vi "Remove Attribute - Many.vi"(8 "error in (no error)":errorcluster, 10 "Attributes":string[](array[string]), 11 "YAML Parser in":refnum<class "YAML Parser.lvclass">) -> (0 "error out":errorcluster, 2 "All Found":bool, 3 "YAML Parser out":refnum<class "YAML Parser.lvclass">)   [LabVIEW 2015, in "YAML Parser.lvclass"]
uses:
  YAML Parser.lvclass
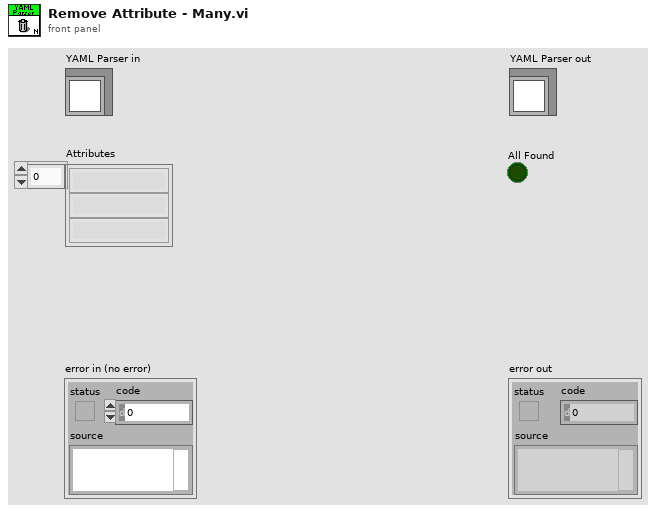
[diagram p1: front panel]
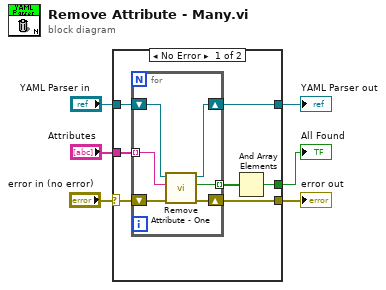
[diagram p0: block diagram]
diagram:
  n1 = case shown="No Error" "error in (no error)" {
    selector: "error in (no error)" -> [w13 w21]
    tunnel: [w12 w21] -> w5
    tunnel: [w10 w20] -> w3
    tunnel: "YAML Parser in" -> [w11 w20]
    tunnel: "Attributes" -> [w9 _]
    tunnel: [w7 _] -> w1
    frame No Error {
      n2 = for {
        tunnel: w9 -> [w15] mode=indexing
        shift-right: [w18] -> w12
        shift-left: w13 -> [w19]
        shift-right: [w16] -> w10
        shift-left: w11 -> [w17]
        tunnel: [w14] -> w8 mode=indexing
        n3 = call "Remove Attribute - One.vi"("error in (no error)"=w19, "Attribute"=w15, "YAML Parser in"=w17) -> ("error out"=w18:errorcluster, "found"=w14:bool, "YAML Parser out"=w16:refnum<class "YAML Parser.lvclass">)  [unwired: 6 in]
      }
      n4 = And Array Elements(Boolean array=w8) -> (logical AND=w7:bool)
    }
    frame Error {
    }
  }
  "error out" <- w5
  "YAML Parser out" <- w3
  "All Found" <- w1
